vi "PQexec.vi"(0 "conn":u32, 1 "query":string, 2 "error in (no error)":errorcluster) -> (4 "PGresult":u32, 6 "error out":errorcluster)   [LabVIEW 2018, in "libpqlv.lvlib"]
doc: "Submits a command to the server and waits for the result.\nReturns a PGresult pointer or possibly a null pointer. A non-null pointer will generally be returned except in out-of-memory conditions or serious errors such as inability to send the command to the server. If a null pointer is returned, it should be treated like a PGRES_FATAL_ERROR result. Use PQerrorMessage to get more information about such errors.\nhttp://www.postgresql.org/docs/8.3/static/libpq-exec.html"
uses:
  libpqlv.lvlib
  lib/libpq.dll
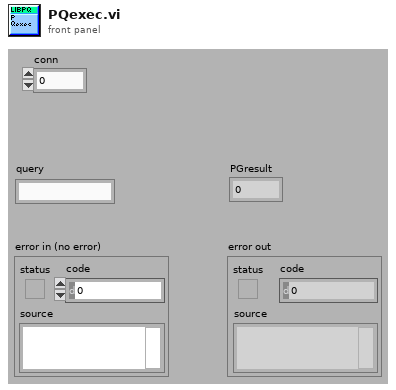
[diagram p1: front panel]
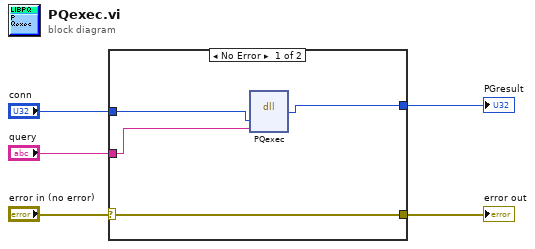
[diagram p0: block diagram]
diagram:
  n1 = case shown="No Error" "error in (no error)" {
    selector: "error in (no error)" -> [w9 w10]
    tunnel: [w9 w10] -> w4
    tunnel: [w8 _] -> w3
    tunnel: "query" -> [w7 _]
    tunnel: "conn" -> [w6 _]
    frame No Error {
      n2 = dll-call lib="D:/Users/erics/Documents/TC-3/DAQ/PostgreSQL2LabVIEW/libpqlv/lib/libpq.*" fn="PQexec"("conn"=w6, "query"=w7) -> ("PGresult"=w8:u32)  [unwired: 5 in, 2 out]
    }
    frame Error {
    }
  }
  "PGresult" <- w3
  "error out" <- w4
